vi "Pulse Measurements N chan (obs).vi"(6 "percent level settings":T3={"method"=enum."auto select", "histogram size"=256, "histogram method"=enum."mode", "reserved"=1.0} {"reserved" format="%0.2f"}, 7 "pulse number (1)":i32=1 min=1, 8 "error in (no error)":errorcluster, 9 "reference levels":T2={"high ref level"=90.0, "mid ref level"=50.0, "low ref level"=10.0, "ref units"=1} {"ref units" items=["absolute", "percent"]; "high ref level" format="%.2p"; "low ref level" format="%.2p"; "mid ref level" format="%.2p"}, 10 "polarity (high)":u16(ring)=1 items=["low pulse", "high pulse"], 11 "signal(s) in":waveform(dbl)[](array[waveform])) -> (0 "error out":errorcluster, 1 "duty cycle":dbl[](array[numeric]) format="%.2p", 2 "pulse duration":dbl[](array[numeric]) format="%.2p", 3 "period":dbl[](array[numeric]) format="%.2p", 4 "measurement info":T1(array[cluster]))   [LabVIEW 2020, in "NI_MAPro.lvlib"]
uses:
  NI_MAPro.lvlib
  NI_MABase.lvlib
panel:
  # "This VI is obsolete !!!\nYou should replace this VI in your diagram with the Pulse Measurements VI."
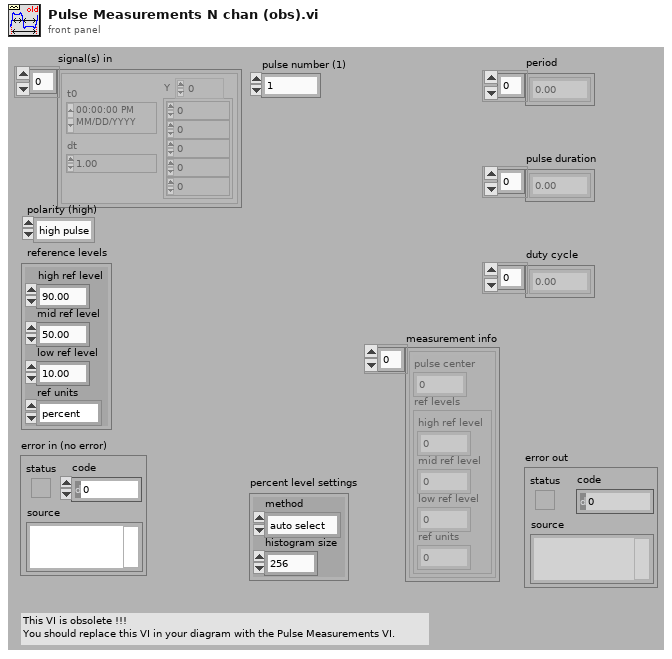
[diagram p1: front panel]
types:
  T1 = cluster{"pulse center":dbl, "ref levels":cluster{"high ref level":dbl, "mid ref level":dbl, "low ref level":dbl, "ref units":u16}}[]
  T2 = cluster{"high ref level":dbl, "mid ref level":dbl, "low ref level":dbl, "ref units":u16}
  T3 = cluster{"method":enum32{"histogram", "peak", "auto select"}, "histogram size":i32, "histogram method":enum16{"mode"}, "reserved":dbl}
  T4 = cluster{"pulse center":dbl, "ref levels":cluster{"high ref level":dbl, "mid ref level":dbl, "low ref level":dbl, "ref units":u16}}
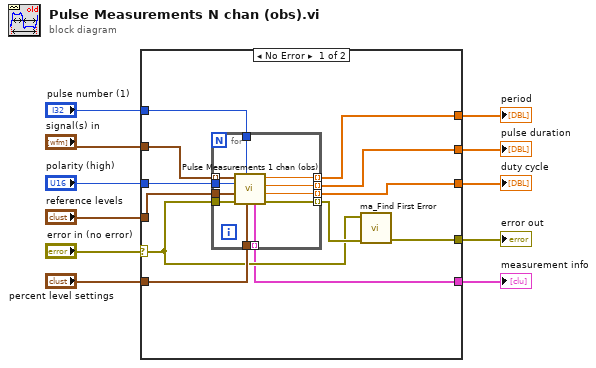
[diagram p0: block diagram]
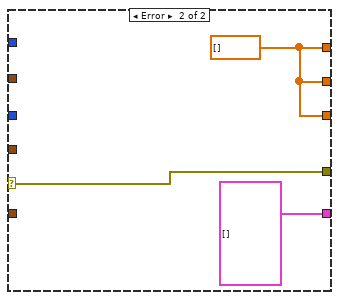
[diagram p2: hidden frame]
diagram:
  n1 = case shown="No Error" "error in (no error)" {
    selector: "error in (no error)" -> [w17 w37]
    tunnel: "percent level settings" -> [w22 _]
    tunnel: [w16 w37] -> w9
    tunnel: "signal(s) in" -> [w23 _]
    tunnel: [w21 w35] -> w7
    tunnel: [w20 w35] -> w6
    tunnel: [w19 w35] -> w5
    tunnel: "reference levels" -> [w15 _]
    tunnel: "pulse number (1)" -> [w14 _]
    tunnel: "polarity (high)" -> [w13 _]
    tunnel: [w12 T1 []] -> w1
    frame No Error {
      n2 = for {
        tunnel: w17 -> [w34]
        tunnel: w22 -> [w33]
        tunnel: [w32] -> w18 mode=indexing
        tunnel: [w31] -> w21 mode=indexing
        tunnel: [w30] -> w20 mode=indexing
        tunnel: [w29] -> w19 mode=indexing
        tunnel: w23 -> [w28] mode=indexing
        tunnel: w15 -> [w27]
        tunnel: w14 -> [w26]
        tunnel: w13 -> [w25]
        tunnel: [w24] -> w12 mode=indexing
        n3 = call "Pulse Measurements 1 chan (obs).vi"("percent level settings"=w33, "pulse number (1)"=w26, "error in (no error)"=w34, "reference levels"=w27, "polarity (high)"=w25, "signal in"=w28) -> ("error out"=w32:errorcluster, "duty cycle"=w29:dbl, "pulse duration"=w30:dbl, "period"=w31:dbl, "measurement info"=w24:T4)  [unwired: 1 out]
      }
      n4 = call "ma_Find First Error.vi"("error array in"=w18, "error in 1 (no error)"=w17) -> ("error out"=w16:errorcluster)  [unwired: 2 in, 3 out]
    }
    frame Error {
      w35 = dbl[] []
    }
  }
  "error out" <- w9
  "period" <- w7
  "pulse duration" <- w6
  "duty cycle" <- w5
  "measurement info" <- w1
